vi "Globals.vi"() -> ()   [LabVIEW 2020, in "Application.lvlib"]
uses:
  Data Manager/Data Manager.lvclass
  Application.lvlib
panel:
  out "Data Manager":refnum<class "Data Manager.lvclass">
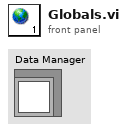
[diagram p1: front panel]
diagram:
